vi "6.0.0_Pump Motor Test.vi"(6 ".batCMD":T1={"Brush_ADC.bat"="Brush_ADC.bat", "Get Release Version.bat"="Get Release Version.bat", "Getting Software  Version.bat"="Getting Software  Version.bat", "Pump_ADC.bat"="Pump_ADC.bat", "Starting  Pump Motor.bat"="Starting  Pump Motor.bat", "Starting  Test Mode.bat"="Starting  Test Mode.bat", "Starting Brush Motor 1.bat"="Starting Brush Motor 1.bat", "Starting Brush Motor 2.bat"="Starting Brush Motor 2.bat", "Starting Brush Motor 3.bat"="Starting Brush Motor 3.bat", "Starting LED Test.bat"="Starting LED Test.bat", "Stopping  Brush Motor.bat"="Stopping  Brush Motor.bat", "Stopping  Pump Motor.bat"="Stopping  Pump Motor.bat", "Stopping  Test Mode.bat"="Stopping  Test Mode.bat", "Starting Self Test.bat"="Starting Self Test.bat", "Software Reset.bat"="Software Reset.bat", "Get HW version.bat"="Get HW version.bat", "Read PMIC status.bat"="Read PMIC status.bat", "SC IMU Data Streaming.bat"="SC IMU Data Streaming.bat"}, 7 "Data in":T2, 8 "error in (no error)":errorcluster, 9 "AllControls In":T3, 10 "?":T4, 11 "Message Queue out":T5) -> (0 "error out":errorcluster, 1 "Flow":string, 2 "Data":T4, 3 "Message Queue Out":T5, 5 "Data out":T2)   [LabVIEW 2017]
uses:
  Depends/AMC/subVIs/TypeDefs/amc_Message Queue.ctl
  Depends/AMC/subVIs/TypeDefs/amc_Message.ctl
  Depends/Tools/Keyed Array/Tools_KeyedArray KeyedArray.ctl
  Ctrls/Data.ctl
  Ctrls/AllControls.ctl
  Ctrls/CSV_Data.ctl
  0516/X682 Chassis Connectivity Tester Program/Ctrls/682_cmd.ctl
  <instrlib>/GPP/GPP.lvlib
types:
  T1 = typedef "682_cmd.ctl" = cluster{"Brush_ADC.bat":string, "Get Release Version.bat":string, "Getting Software  Version.bat":string, "Pump_ADC.bat":string, "Starting  Pump Motor.bat":string, "Starting  Test Mode.bat":string, "Starting Brush Motor 1.bat":string, "Starting Brush Motor 2.bat":string, "Starting Brush Motor 3.bat":string, "Starting LED Test.bat":string, "Stopping  Brush Motor.bat":string, "Stopping  Pump Motor.bat":string, "Stopping  Test Mode.bat":string, "Starting Self Test.bat":string, "Software Reset.bat":string, "Get HW version.bat":string, "Read PMIC status.bat":string, "SC IMU Data Streaming.bat":string}
  T2 = typedef "CSV_Data.ctl" = cluster{"Initialisation":cluster{"LMT - Connect UUT (con COM)":string, "LMT - Software Version (rrel)":string, "LMT - Write SKU file (wskuc)":string, "LMT - SKU file name":string, "Connect UUT DDM":string, "Read DDM EOL Timestamp - Mode":string, "Read DDM EOL Timestamp - Timestamp":string, "Read DDM EOL Timestamp - Rig ID":string, "Read DDM EOL Timestamp - Passmark ID":string, "Read DDM EOL Timestamp - Passmark Rev":string, "Software Version before flashing":string, "Read Hardware Serial":string, "UUT DDM SN":string, "Compare DDM SN with MES SN":string, "Backup PCBA Calibration EEPROM Response - CAL":string, "Flash Firmware Version":string, "Check SW Version":string, "Read DDM SW Version after flashing":string, "Set SKU Config":string, "Ready Status":string, "Set Device Mode to EOL":string, "DDM Parameter - Voltage":string, "DDM Parameter - Current":string, "DDM Parameter - Power":string, "DDM Parameter - Speed":string, "DDM Parameter - Pressure":string, "Tester Parameter - Voltage":string, "Tester Parameter - Current":string, "Tester Parameter - Power":string, "Tester Parameter - Ambient Pressure":string, "Tester Parameter - Ambient Temperature":string, "Calculated Parameter - DDM Pressure Corrected":string, "Calculated Parameter - DDM Real Power":string, "Calculated Parameter - Delta V":string}, "BEMF_Calibration":cluster{"Calibration Result - eol_cold_bemf_temp":string, "DDM Ambient Temp":string, "Restriction Plate Diameter":string, "Calibration Result - eol_bemf_mp_cold_coef_a":string, "Calibration Result - eol_bemf_mp_cold_coef_b":string, "Calibration Result - eol_bemf_mp_cold_coef_c":string, "Calibration Result - eol_bemf_lsi_cold_ref_coeffs":string, "Get - Calibration Result - eol_bemf_lsi_speed":string, "Get - Calibration Result - eol_bemf_lsi_integral_0":string, "Calibration Result - eol_bemf_lsi_integral_1":string, "Get - Calibration Result - eol_bemf_lsi_integral_2":string, "Get - Calibration Result - eol_cold_bemf":string, "Get - Calibration Result - eol_cold_bemf_fisf":string, "Finalise Calibration":string, "Compare -Calibration Result - eol_cold_bemf":string, "Compare -Calibration Result - eol_cold_bemf_fisf":string}, "ECO":cluster{"Reset Power Tune":string, "Reset BEMF FISF Calibration":string, "Restriction Plate Diameter":string, "ECO - Stabilisation Time":string, "ECO - DDM Parameter - Voltage":string, "ECO - DDM Parameter - Current":string, "ECO - DDM Parameter - Power":string, "ECO - DDM Parameter - Measured Power":string, "ECO - DDM Parameter - Speed":string, "ECO - DDM Parameter - Pressure":string, "ECO - Tester Parameter - Voltage":string, "ECO - Tester Parameter - Current":string, "ECO - Tester Parameter - Power":string, "ECO - Tester Parameter - Ambient Pressure":string, "ECO - Tester Parameter - Ambient Temperature":string, "ECO - Tester Parameter - Ambient Humidity":string, "ECO - Calculated Parameter - DDM Pressure Corrected":string, "ECO - Calculated Parameter - DDM Real Power":string, "ECO - Calculated Parameter - Delta V":string, "ECO - Calculated Parameter - Flowrate":string, "ECO - Calculated Parameter - Airwatt":string, "ECO - Formula":string, "PT ECO - Power Tune Mode Status":string}, "BOOST":cluster{"Restriction Plate Diameter":string, "BOOST - Stabilisation Time":string, "BOOST - DDM Parameter - Voltage":string, "BOOST - DDM Parameter - Current":string, "BOOST - DDM Parameter - Power":string, "BOOST - DDM Parameter - Measured Power":string, "BOOST - DDM Parameter - Speed":string, "BOOST - DDM Parameter - Pressure":string, "BOOST - Tester Parameter - Voltage":string, "BOOST - Tester Parameter - Current":string, "BOOST - Tester Parameter - Power":string, "BOOST - Tester Parameter - Ambient Pressure":string, "BOOST - Tester Parameter - Ambient Temperature":string, "BOOST - Tester Parameter - Ambient Humidity":string, "BOOST - Calculated Parameter - DDM Pressure Corrected":string, "BOOST - Calculated Parameter - DDM Real Power":string, "BOOST - Calculated Parameter - Delta V":string, "BOOST - Calculated Parameter - Flowrate":string, "BOOST - Calculated Parameter - Airwatt":string, "BOOST - Get AM Presence":string, "Air Muscle Turn Off Status":string, "BOOST - Air Muscle Calculated Parameter - Airwatt B":string, "BOOST - Air Muscle Calculate Airwatt Delta":string, "PT BOOST - Power Tune Mode Status":string, "Finalise Calibration":string, "ECO - Get AW Calibration value":string, "BOOST - Get AW Calibration value":string}, "MAX":cluster{"Restriction Plate Diameter":string, "MAX - Stabilisation Time":string, "Get Average Delta Tmag (LSIdelta_FISFdelta_LSItmag_FISFtmag_IIRtmag)":string, "Get Average Delta Tmag FISF":string, "MAX - DDM Parameter - Voltage":string, "MAX - DDM Parameter - Current":string, "MAX - DDM Parameter - Power":string, "MAX - DDM Parameter - Measured Power":string, "MAX - DDM Parameter - Speed":string, "MAX - DDM Parameter - Pressure":string, "MAX - Tester Parameter - Voltage":string, "MAX - Tester Parameter - Current":string, "MAX - Tester Parameter - Power":string, "MAX - Tester Parameter - Ambient Pressure":string, "MAX - Tester Parameter - Ambient Temperature":string, "MAX - Tester Parameter - Ambient Humidity":string, "MAX - Calculated Parameter - DDM Pressure Corrected":string, "MAX - Calculated Parameter - DDM Real Power":string, "MAX - Calculated Parameter - Delta V":string, "MAX - Calculated Parameter - Flowrate":string, "MAX - Calculated Parameter - Airwatt":string, "MAX_FISF_Check_Average_Delta_Tmag":string, "MAX - FISF - BEMF Finetune Result":string, "MAX tune - Delta P1":string, "MAX tune - Calculated Parameter - Airwatt":string, "Calculate Delta Airwatts - MAX finetune - Delta P2":string, "MAX finetune - DDM Parameter - Voltage":string, "MAX finetune - DDM Parameter - Current":string, "MAX finetune - DDM Parameter - Power":string, "MAX finetune - DDM Parameter - Measured Power":string, "MAX finetune - DDM Parameter - Speed":string, "MAX finetune - DDM Parameter - Pressure":string, "MAX finetune - Tester Parameter - Voltage":string, "MAX finetune - Tester Parameter - Current":string, "MAX finetune - Tester Parameter - Power":string, "MAX finetune - Tester Parameter - Ambient Pressure":string, "MAX finetune - Tester Parameter - Ambient Temperature":string, "MAX finetune - Tester Parameter - Ambient Humidity":string, "MAX finetune - Calculated Parameter - DDM Pressure Corrected":string, "MAX finetune - Calculated Parameter - DDM Real Power":string, "MAX finetune - Calculated Parameter - Delta V":string, "MAX finetune - Calculated Parameter - Flowrate":string, "MAX finetune - Calculated Parameter - Airwatt":string, "Check Derate Result":string, "Delta Tmag FISF":string, "Get Hot BEMF Result":string, "Calculate delta Pressure":string, "Finalise Calibration":string, "Calculate & Check Delta BEMF":string, "Delta P Airwatts Value":string}, "LL":cluster{"DDM Ambient Temp":string, "Restriction Plate Diameter":string, "LL - DDM Parameter - Voltage":string, "LL - DDM Parameter - Current":string, "LL - DDM Parameter - Power":string, "LL - DDM Parameter - Measured Power":string, "LL - DDM Parameter - Speed":string, "LL - DDM Parameter - Pressure":string, "LL - Tester Parameter - Voltage":string, "LL - Tester Parameter - Current":string, "LL - Tester Parameter - Power":string, "LL - DDM Real Power":string, "LL - Calibrate Task Detect LL":string}, "HL":cluster{"HL - DDM Parameter - Voltage":string, "HL - DDM Parameter - Current":string, "HL - DDM Parameter - Power":string, "HL - DDM Parameter - Measured Power":string, "HL - DDM Parameter - Speed":string, "HL - DDM Parameter - Pressure":string, "HL - Tester Parameter - Voltage":string, "HL - Tester Parameter - Current":string, "HL - Tester Parameter - Power":string, "HL - DDM Real Power":string, "HL - Calibrate Task Detect HL":string}, "LH":cluster{"Restriction Plate Diameter":string, "LH - DDM Parameter - Voltage":string, "LH - DDM Parameter - Current":string, "LH - DDM Parameter - Power":string, "LH - DDM Parameter - Measured Power":string, "LH - DDM Parameter - Speed":string, "LH - DDM Parameter - Pressure":string, "LH - Tester Parameter - Voltage":string, "LH - Tester Parameter - Current":string, "LH - Tester Parameter - Power":string, "LH - DDM Real Power":string, "LH - Calibrate Task Detect LH":string}, "HH":cluster{"HH - DDM Parameter - Voltage":string, "HH - DDM Parameter - Current":string, "HH - DDM Parameter - Power":string, "HH - DDM Parameter - Measured Power":string, "HH - DDM Parameter - Speed":string, "HH - DDM Parameter - Pressure":string, "HH - Tester Parameter - Voltage":string, "HH - Tester Parameter - Current":string, "HH - Tester Parameter - Power":string, "HH - DDM Real Power":string, "HH - Calibrate Task Detect HH":string}, "Inlet Blockage Calibration":cluster{"Inlet Blockage Calibration - DDM Parameter - Voltage":string, "Inlet Blockage Calibration - DDM Parameter - Current":string, "Inlet Blockage Calibration - DDM Parameter - Power":string, "Inlet Blockage Calibration - DDM Parameter - Measured Power":string, "Inlet Blockage Calibration - DDM Parameter - Speed":string, "Inlet Blockage Calibration - DDM Parameter - Pressure":string, "Inlet Blockage Calibration - Tester Parameter - Voltage":string, "Inlet Blockage Calibration - Tester Parameter - Current":string, "Inlet Blockage Calibration - Tester Parameter - Power":string, "Inlet Blockage Calibration - DDM Real Power":string, "Calibration Inlet Blockage_E":string, "Finalise Calibration":string, "Get Task Detect LL":string, "Get Task Detect HL":string, "Get Task Detect LH":string, "Get Task Detect HH":string, "Calibration Inlet Blockage":string, "Calibration eol cold bemf temp":string}, "GOOD":cluster{"GOOD UNIT - Clear EEPROM Error Log":string, "GOOD UNIT - Write Product Timestamp - Mode":string, "GOOD UNIT - Write Product Timestamp - Timestamp":string, "GOOD UNIT - Write Product Timestamp - Rig ID":string, "GOOD UNIT - Write Product Timestamp - Passmark ID":string, "GOOD UNIT - Write Product Timestamp - Passmark Rev":string, "GOOD UNIT - Set Device Mode to PROD":string, "GOOD UNIT - Backup PCBA Calibration EEPROM Response":string, "GOOD UNIT - Check Security Bit":string, "GOOD UNIT - Set Calibration Lock":string, "GOOD UNIT - Get_Calibration_Lock":string, "GOOD UNIT - Disconnect UUT":string}, "NG":cluster{"NG UNIT - Read NVM Error":string, "NG UNIT - Set Device Mode to FCT":string, "NG UNIT - Backup PCBA Calibration EEPROM Response - CAL":string, "NG UNIT - Backup PCBA Calibration EEPROM Response - ERROR":string, "NG UNIT - Backup PCBA Calibration EEPROM Response - USAGE":string, "NG UNIT - Disconnect UUT":string}, "SN":string, "Table":string[][], "Count":cluster{"Total":i32, "OK":i32, "NG":i32, "Yield":dbl}, "Start Time":timestamp, "daemon reference":refnum<k5>, "CT":dbl, "Config":string[][], "OK/NG":bool, "Station ID":string, "MES DDM SN":string, "MES PCBA SN":string, "Retest":string, "Lux":string, "Initialisation_Status":cluster{"LMT - Connect UUT (con COM)":string, "LMT - Software Version (rrel)":string, "LMT - Write SKU file (wskuc)":string, "LMT - SKU file name":string, "Connect UUT DDM":string, "Read DDM EOL Timestamp - Mode":string, "Read DDM EOL Timestamp - Timestamp":string, "Read DDM EOL Timestamp - Rig ID":string, "Read DDM EOL Timestamp - Passmark ID":string, "Read DDM EOL Timestamp - Passmark Rev":string, "Software Version before flashing":string, "Read Hardware Serial":string, "UUT DDM SN":string, "Compare DDM SN with MES SN":string, "Backup PCBA Calibration EEPROM Response - CAL":string, "Flash Firmware Version":string, "Check SW Version":string, "Read DDM SW Version after flashing":string, "Set SKU Config":string, "Ready Status":string, "Set Device Mode to EOL":string, "DDM Parameter - Voltage":string, "DDM Parameter - Current":string, "DDM Parameter - Power":string, "DDM Parameter - Speed":string, "DDM Parameter - Pressure":string, "Tester Parameter - Voltage":string, "Tester Parameter - Current":string, "Tester Parameter - Power":string, "Tester Parameter - Ambient Pressure":string, "Tester Parameter - Ambient Temperature":string, "Calculated Parameter - DDM Pressure Corrected":string, "Calculated Parameter - DDM Real Power":string, "Calculated Parameter - Delta V":string}, "BEMF_Calibration_Status":cluster{"Calibration Result - eol_cold_bemf_temp":string, "DDM Ambient Temp":string, "Restriction Plate Diameter":string, "Calibration Result - eol_bemf_mp_cold_coef_a":string, "Calibration Result - eol_bemf_mp_cold_coef_b":string, "Calibration Result - eol_bemf_mp_cold_coef_c":string, "Calibration Result - eol_bemf_lsi_cold_ref_coeffs":string, "Get - Calibration Result - eol_bemf_lsi_speed":string, "Get - Calibration Result - eol_bemf_lsi_integral_0":string, "Calibration Result - eol_bemf_lsi_integral_1":string, "Get - Calibration Result - eol_bemf_lsi_integral_2":string, "Get - Calibration Result - eol_cold_bemf":string, "Get - Calibration Result - eol_cold_bemf_fisf":string, "Finalise Calibration":string, "Compare -Calibration Result - eol_cold_bemf":string, "Compare -Calibration Result - eol_cold_bemf_fisf":string}, "ECO_Status":cluster{"Reset Power Tune":string, "Reset BEMF FISF Calibration":string, "Restriction Plate Diameter":string, "ECO - Stabilisation Time":string, "ECO - DDM Parameter - Voltage":string, "ECO - DDM Parameter - Current":string, "ECO - DDM Parameter - Power":string, "ECO - DDM Parameter - Measured Power":string, "ECO - DDM Parameter - Speed":string, "ECO - DDM Parameter - Pressure":string, "ECO - Tester Parameter - Voltage":string, "ECO - Tester Parameter - Current":string, "ECO - Tester Parameter - Power":string, "ECO - Tester Parameter - Ambient Pressure":string, "ECO - Tester Parameter - Ambient Temperature":string, "ECO - Tester Parameter - Ambient Humidity":string, "ECO - Calculated Parameter - DDM Pressure Corrected":string, "ECO - Calculated Parameter - DDM Real Power":string, "ECO - Calculated Parameter - Delta V":string, "ECO - Calculated Parameter - Flowrate":string, "ECO - Calculated Parameter - Airwatt":string, "ECO - Formula":string, "PT ECO - Power Tune Mode Status":string}, "BOOST_Status":cluster{"Restriction Plate Diameter":string, "BOOST - Stabilisation Time":string, "BOOST - DDM Parameter - Voltage":string, "BOOST - DDM Parameter - Current":string, "BOOST - DDM Parameter - Power":string, "BOOST - DDM Parameter - Measured Power":string, "BOOST - DDM Parameter - Speed":string, "BOOST - DDM Parameter - Pressure":string, "BOOST - Tester Parameter - Voltage":string, "BOOST - Tester Parameter - Current":string, "BOOST - Tester Parameter - Power":string, "BOOST - Tester Parameter - Ambient Pressure":string, "BOOST - Tester Parameter - Ambient Temperature":string, "BOOST - Tester Parameter - Ambient Humidity":string, "BOOST - Calculated Parameter - DDM Pressure Corrected":string, "BOOST - Calculated Parameter - DDM Real Power":string, "BOOST - Calculated Parameter - Delta V":string, "BOOST - Calculated Parameter - Flowrate":string, "BOOST - Calculated Parameter - Airwatt":string, "BOOST - Get AM Presence":string, "Air Muscle Turn Off Status":string, "BOOST - Air Muscle Calculated Parameter - Airwatt B":string, "BOOST - Air Muscle Calculate Airwatt Delta":string, "PT BOOST - Power Tune Mode Status":string, "Finalise Calibration":string, "ECO - Get AW Calibration value":string, "BOOST - Get AW Calibration value":string}, "MAX_Status":cluster{"Restriction Plate Diameter":string, "MAX - Stabilisation Time":string, "Get Average Delta Tmag (LSIdelta_FISFdelta_LSItmag_FISFtmag_IIRtmag)":string, "Get Average Delta Tmag FISF":string, "MAX - DDM Parameter - Voltage":string, "MAX - DDM Parameter - Current":string, "MAX - DDM Parameter - Power":string, "MAX - DDM Parameter - Measured Power":string, "MAX - DDM Parameter - Speed":string, "MAX - DDM Parameter - Pressure":string, "MAX - Tester Parameter - Voltage":string, "MAX - Tester Parameter - Current":string, "MAX - Tester Parameter - Power":string, "MAX - Tester Parameter - Ambient Pressure":string, "MAX - Tester Parameter - Ambient Temperature":string, "MAX - Tester Parameter - Ambient Humidity":string, "MAX - Calculated Parameter - DDM Pressure Corrected":string, "MAX - Calculated Parameter - DDM Real Power":string, "MAX - Calculated Parameter - Delta V":string, "MAX - Calculated Parameter - Flowrate":string, "MAX - Calculated Parameter - Airwatt":string, "MAX_FISF_Check_Average_Delta_Tmag":string, "MAX - FISF - BEMF Finetune Result":string, "MAX tune - Delta P1":string, "MAX tune - Calculated Parameter - Airwatt":string, "Calculate Delta Airwatts - MAX finetune - Delta P2":string, "MAX finetune - DDM Parameter - Voltage":string, "MAX finetune - DDM Parameter - Current":string, "MAX finetune - DDM Parameter - Power":string, "MAX finetune - DDM Parameter - Measured Power":string, "MAX finetune - DDM Parameter - Speed":string, "MAX finetune - DDM Parameter - Pressure":string, "MAX finetune - Tester Parameter - Voltage":string, "MAX finetune - Tester Parameter - Current":string, "MAX finetune - Tester Parameter - Power":string, "MAX finetune - Tester Parameter - Ambient Pressure":string, "MAX finetune - Tester Parameter - Ambient Temperature":string, "MAX finetune - Tester Parameter - Ambient Humidity":string, "MAX finetune - Calculated Parameter - DDM Pressure Corrected":string, "MAX finetune - Calculated Parameter - DDM Real Power":string, "MAX finetune - Calculated Parameter - Delta V":string, "MAX finetune - Calculated Parameter - Flowrate":string, "MAX finetune - Calculated Parameter - Airwatt":string, "Check Derate Result":string, "Delta Tmag FISF":string, "Get Hot BEMF Result":string, "Calculate delta Pressure":string, "Finalise Calibration":string, "Calculate & Check Delta BEMF":string, "Delta P Airwatts Value":string}, "LL_Status":cluster{"DDM Ambient Temp":string, "Restriction Plate Diameter":string, "LL - DDM Parameter - Voltage":string, "LL - DDM Parameter - Current":string, "LL - DDM Parameter - Power":string, "LL - DDM Parameter - Measured Power":string, "LL - DDM Parameter - Speed":string, "LL - DDM Parameter - Pressure":string, "LL - Tester Parameter - Voltage":string, "LL - Tester Parameter - Current":string, "LL - Tester Parameter - Power":string, "LL - DDM Real Power":string, "LL - Calibrate Task Detect LL":string}, "HL_Status":cluster{"HL - DDM Parameter - Voltage":string, "HL - DDM Parameter - Current":string, "HL - DDM Parameter - Power":string, "HL - DDM Parameter - Measured Power":string, "HL - DDM Parameter - Speed":string, "HL - DDM Parameter - Pressure":string, "HL - Tester Parameter - Voltage":string, "HL - Tester Parameter - Current":string, "HL - Tester Parameter - Power":string, "HL - DDM Real Power":string, "HL - Calibrate Task Detect HL":string}, "LH_Status":cluster{"Restriction Plate Diameter":string, "LH - DDM Parameter - Voltage":string, "LH - DDM Parameter - Current":string, "LH - DDM Parameter - Power":string, "LH - DDM Parameter - Measured Power":string, "LH - DDM Parameter - Speed":string, "LH - DDM Parameter - Pressure":string, "LH - Tester Parameter - Voltage":string, "LH - Tester Parameter - Current":string, "LH - Tester Parameter - Power":string, "LH - DDM Real Power":string, "LH - Calibrate Task Detect LH":string}, "HH_Status":cluster{"HH - DDM Parameter - Voltage":string, "HH - DDM Parameter - Current":string, "HH - DDM Parameter - Power":string, "HH - DDM Parameter - Measured Power":string, "HH - DDM Parameter - Speed":string, "HH - DDM Parameter - Pressure":string, "HH - Tester Parameter - Voltage":string, "HH - Tester Parameter - Current":string, "HH - Tester Parameter - Power":string, "HH - DDM Real Power":string, "HH - Calibrate Task Detect HH":string}, "Inlet Blockage Calibration_Status":cluster{"Inlet Blockage Calibration - DDM Parameter - Voltage":string, "Inlet Blockage Calibration - DDM Parameter - Current":string, "Inlet Blockage Calibration - DDM Parameter - Power":string, "Inlet Blockage Calibration - DDM Parameter - Measured Power":string, "Inlet Blockage Calibration - DDM Parameter - Speed":string, "Inlet Blockage Calibration - DDM Parameter - Pressure":string, "Inlet Blockage Calibration - Tester Parameter - Voltage":string, "Inlet Blockage Calibration - Tester Parameter - Current":string, "Inlet Blockage Calibration - Tester Parameter - Power":string, "Inlet Blockage Calibration - DDM Real Power":string, "Calibration Inlet Blockage_E":string, "Finalise Calibration":string, "Get Task Detect LL":string, "Get Task Detect HL":string, "Get Task Detect LH":string, "Get Task Detect HH":string, "Calibration Inlet Blockage":string, "Calibration eol cold bemf temp":string}, "GOOD_Status":cluster{"GOOD UNIT - Clear EEPROM Error Log":string, "GOOD UNIT - Write Product Timestamp - Mode":string, "GOOD UNIT - Write Product Timestamp - Timestamp":string, "GOOD UNIT - Write Product Timestamp - Rig ID":string, "GOOD UNIT - Write Product Timestamp - Passmark ID":string, "GOOD UNIT - Write Product Timestamp - Passmark Rev":string, "GOOD UNIT - Set Device Mode to PROD":string, "GOOD UNIT - Backup PCBA Calibration EEPROM Response":string, "GOOD UNIT - Check Security Bit":string, "GOOD UNIT - Set Calibration Lock":string, "GOOD UNIT - Get_Calibration_Lock":string, "GOOD UNIT - Disconnect UUT":string}, "NG_Status":cluster{"NG UNIT - Read NVM Error":string, "NG UNIT - Set Device Mode to FCT":string, "NG UNIT - Backup PCBA Calibration EEPROM Response - CAL":string, "NG UNIT - Backup PCBA Calibration EEPROM Response - ERROR":string, "NG UNIT - Backup PCBA Calibration EEPROM Response - USAGE":string, "NG UNIT - Disconnect UUT":string}, "SKU":string, "Plate_Diameter":string, "Alarm":string}
  T3 = typedef "AllControls.ctl" = cluster{"MainVI":refnum<vi>, "AlarmInfo":refnum<vi>, "Log":refnum<vi>, "Current CT":refnum<vi>, "ProductID":refnum<vi>, "Device state":refnum<vi>, "MES":refnum<vi>, "mode":refnum<vi>, "TestInfo":refnum<vi>, "SubPnl":refnum<vi>, "Table":refnum<vi>, "MES bool":refnum<vi>, "TestMode":refnum<vi>, "Recipe":refnum<vi>, "Fail resume":refnum<vi>, "LogIn":refnum<vi>, "Start":refnum<vi>, "Maintenance":refnum<vi>, "Stop":refnum<vi>, "Exit":refnum<vi>}
  T4 = typedef "Data.ctl" = cluster{"Initialisation":cluster{"DDM_Parameter":dbl[], "DDM_Parameter_status":bool[], "Get_Tester_Parameter":dbl[], "Get_Tester_Parameter_status":bool[], "Cal_Tester_Parameter":dbl[], "Cal_Tester_Parameter_status":bool[], "sw_version_before_status":bool, "sw_version_after_status":bool, "Set_SKU_Config_With_LMT_status":bool, "FCT_timestamp_status":bool, "LMT_Connect_to_UUT_status":bool}, "BEMF_Calibration":cluster{"Read_ambient_temperature":dbl, "Calibration_Vaule":dbl[], "Calibration_Vaule _B":dbl[], "Calibration_Vaule_status":bool[], "Calibration_Vaule_B_status":bool[]}, "ECO":cluster{"DDM_Parameter":dbl[], "DDM_Parameter_status":bool[], "Get_Tester_Parameter":dbl[], "Get_Tester_Parameter_status":bool[], "Cal_Tester_Parameter":dbl[], "Cal_Tester_Parameter_status":bool[], "DDM_Parameter_after_power_tune":dbl[], "Get_Tester_Parameter_after_power_tune":dbl[], "Cal_Tester_Parameter_after_power_tune":dbl[], "Cal_Tester_Parameter_after_power_tune_status":bool[], "Delta_P":dbl}, "BOOST":cluster{"DDM_Parameter":dbl[], "DDM_Parameter_status":bool[], "Get_Tester_Parameter":dbl[], "Get_Tester_Parameter_status":bool[], "Cal_Tester_Parameter":dbl[], "Cal_Tester_Parameter_status":bool[], "DDM_Parameter_after_power_tune":dbl[], "Get_Tester_Parameter_after_power_tune":dbl[], "Cal_Tester_Parameter_after_power_tune":dbl[], "Cal_Tester_Parameter_after_power_tune_status":bool[], "airwatts_am_off":dbl, "AW_Delta_(AM_on_and_off)":dbl, "AW_Delta_(AM_on_and_off)_Status":bool, "Delta_P":dbl}, "MAX":cluster{"Average_Tmag_Data":cluster{"LSI Delta in degC":dbl, "FISF Delta in degc":dbl, "LSI Tmag in degC":dbl, "Fisf Tmag in degC":dbl, "IIR Tmag in degC":dbl}, "DDM_Parameter":dbl[], "DDM_Parameter_status":bool[], "Get_Tester_Parameter":dbl[], "Get_Tester_Parameter_status":bool[], "Cal_Tester_Parameter":dbl[], "BEMF_Finetune":cluster{"eol_bemf_mp_cold_coef_c":dbl, "eol_cold_bemf_fisf_offset":dbl}, "AW_Tune":cluster{"delta_P1":dbl, "delta_P_Setting":dbl}, "DDM_Parameter_after_Airwatts_Tune":dbl[], "Get_Tester_Parameter_after_Airwatts_Tune":dbl[], "Cal_Tester_Parameter_after_Airwatts_Tune":dbl[], "DDM_Parameter_after_Airwatts_Finetune":dbl[], "Get_Tester_Parameter_after_Airwatts_Finetune":dbl[], "Cal_Tester_Parameter_after_Airwatts_Finetune":dbl[], "AW_Finetune":cluster{"delta_P2":dbl, "delta_P_Setting":dbl}, "Delta_Tmag_after_tune":cluster{"LSI Delta in degC":dbl, "FISF Delta in degc":dbl, "LSI Tmag in degC":dbl, "Fisf Tmag in degC":dbl, "IIR Tmag in degC":dbl}, "Hot Bemf in mV":dbl, "DDM_Pressure":dbl, "Delta_Pressure":dbl, " Cold Bemf in mV":dbl, " delta Bemf":dbl, " delta p":dbl, "Delta_Pressure_status":bool, " delta Bemf_status":bool, "LSI Delta in degC_status":bool, "FISF Delta in degc_status":bool, "Max_check_derate_status_status":bool, "Average_All_data":dbl[][], "Average_Tmag_Data_status":bool[], "Average_Tmag_Data_after_tune_status":bool[], "Cal_Tester_Parameter_status":bool[], "Cal_Tester_Parameter_status_after_Airwatts_Tune":bool[], "Cal_Tester_Parameter_status_after_Airwatts_FineTune":bool[]}, "Task_Detect_Calib":cluster{"LL":cluster{"DDM_Parameter":dbl[], "DDM_Parameter_status":bool[], "Get_Tester_Parameter":dbl[], "Get_Tester_Parameter_status":bool[], "Set_task_detect_A":dbl, "Set_task_detect_A_Status":bool}, "HL":cluster{"DDM_Parameter":dbl[], "DDM_Parameter_status":bool[], "Get_Tester_Parameter":dbl[], "Get_Tester_Parameter_status":bool[], "Set_task_detect_B":dbl, "Set_task_detect_B_Status":bool}, "LH":cluster{"DDM_Parameter":dbl[], "DDM_Parameter_status":bool[], "Get_Tester_Parameter":dbl[], "Get_Tester_Parameter_status":bool[], "Set_task_detect_C":dbl, "Set_task_detect_C_Status":bool}, "HH":cluster{"DDM_Parameter":dbl[], "DDM_Parameter_status":bool[], "Get_Tester_Parameter":dbl[], "Get_Tester_Parameter_status":bool[], "Set_task_detect_D":dbl, "Read_and_check_calibration_Status":bool[], "Set_task_detect_D_Status":bool}, "Get_eol_inlet_blockage_E":dbl, "Calib_vaule":cluster{"Get_task_detect_LL":dbl, "Get_task_detect_HL":dbl, "Get_task_detect_LH":dbl, "Get_task_detect_HH":dbl, "eol_inlet_blockage":dbl, "eol_code_bemf_temp":dbl}, "calibrated temp":dbl, "Inlet_Blockage_Calibration":cluster{"DDM_Parameter":dbl[], "DDM_Parameter_status":bool[], "Get_Tester_Parameter":dbl[], "Get_Tester_Parameter_status":bool[]}, "Get_eol_inlet_blockage_E_Status":bool}, "good":cluster{"Write_Product_TS":cluster{"TIMESTAMP":i64, "RIG_ID":i64, "PASSMARK_ID":i64, "PASSMARK_REV":i64}, "Read_Product_TS":cluster{"TIMESTAMP":i64, "RIG_ID":i64, "PASSMARK_ID":i64, "PASSMARK_REV":i64}, "Good_Check_Secuity_Bit_Stauts":bool}}
  T5 = typedef "amc_Message Queue.ctl" = refnum<queue>
  T6 = typedef "HD Config.ctl" = cluster{" PC":cluster{"PC Address":u8[], "PC Port":i32}, "FCO":cluster{"COM":refnum<visa-resource-name>, "Baudrate":u32}, "DC Power ":cluster{"COM":refnum<visa-resource-name>, "Baudrate":u32}, "PW3336":cluster{"COM":refnum<visa-resource-name>, "Baudrate":u32}, "Lefoo":cluster{"COM":refnum<visa-resource-name>, "Baudrate":u32}, "Tempt&Hum":cluster{"COM":refnum<visa-resource-name>, "Baudrate":u32}, "DIPC":cluster{"COM":refnum<visa-resource-name>}, "Daemon":cluster{"IP Address":string, "Port":u16, "Retry":u16}, "URAT":cluster{"COM":refnum<visa-resource-name>, "Baudrate":u32}, "Fail_resume_mode":bool, "GRR":bool}
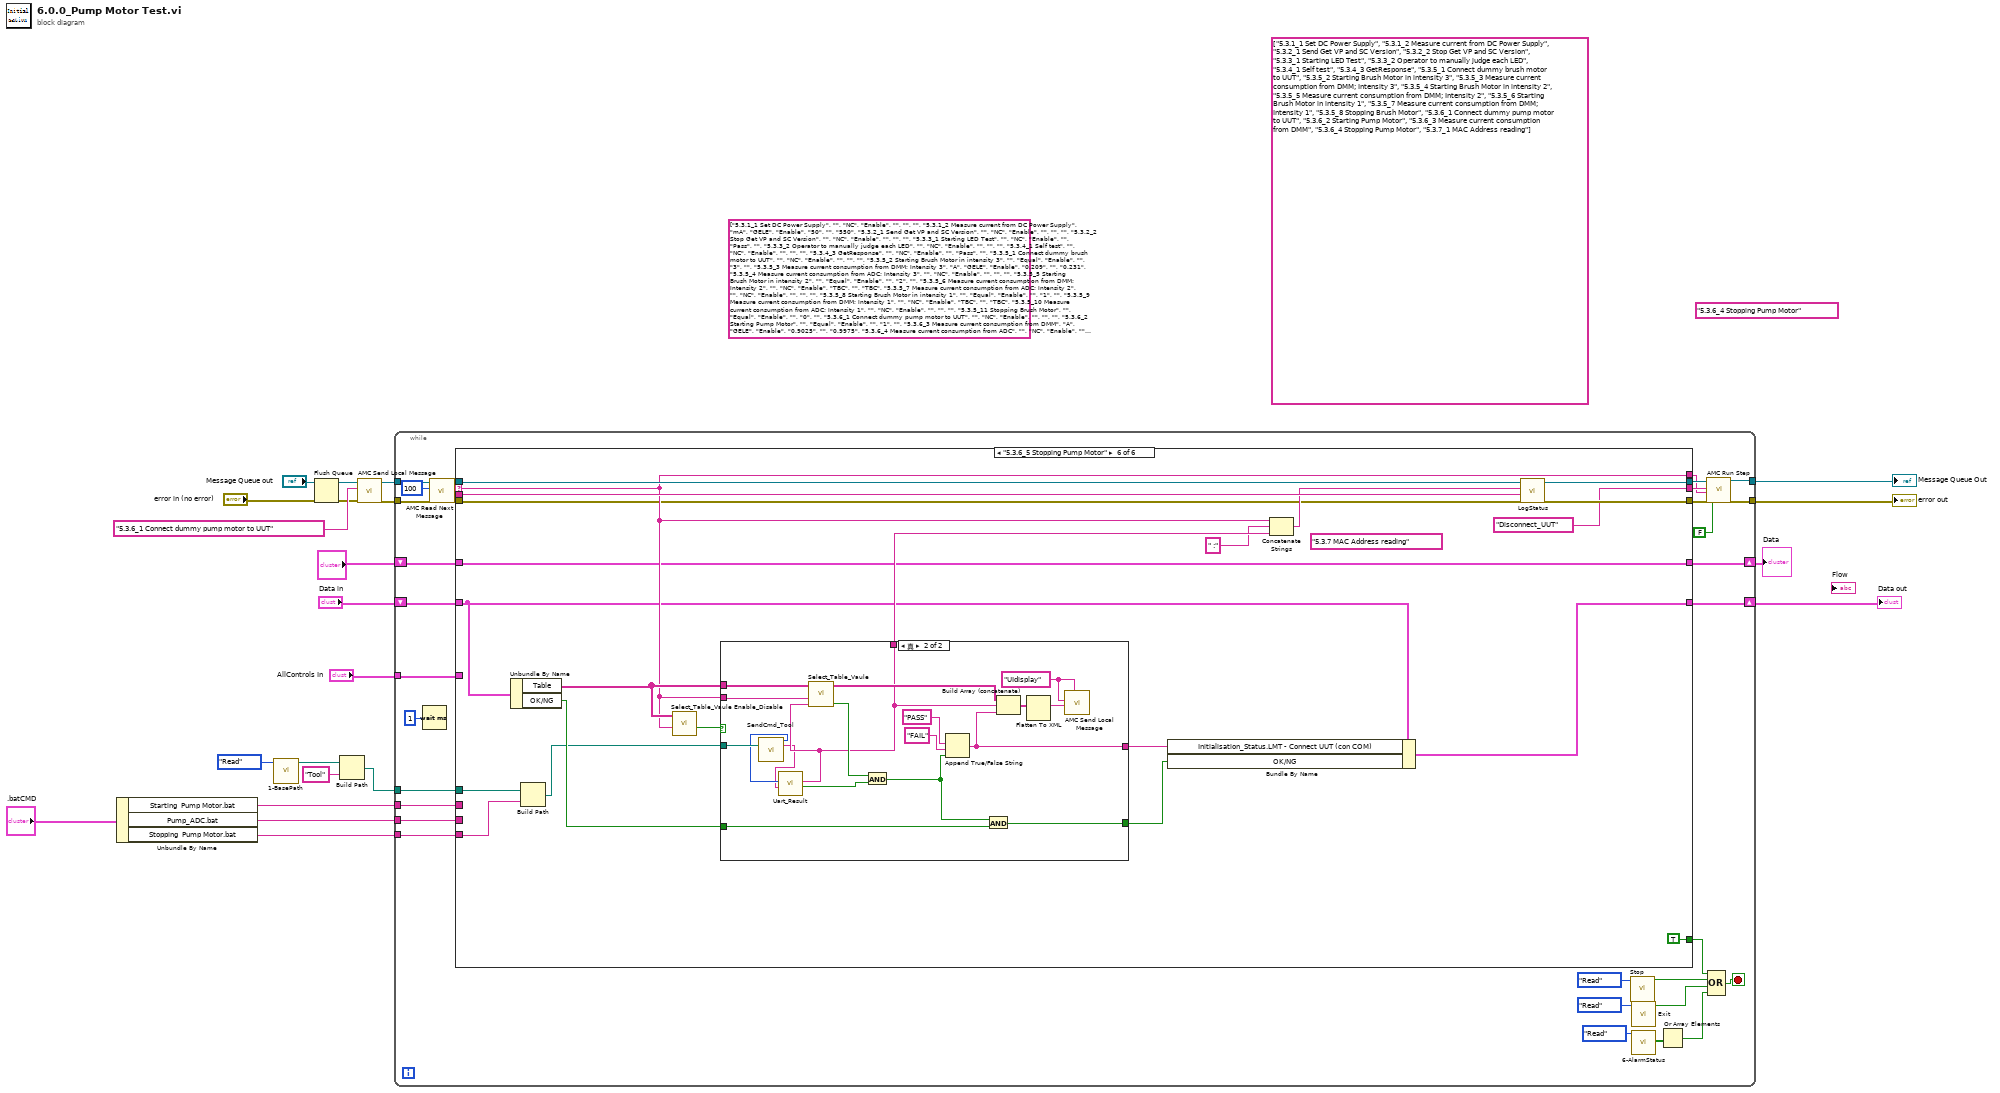
[diagram p0: block diagram]
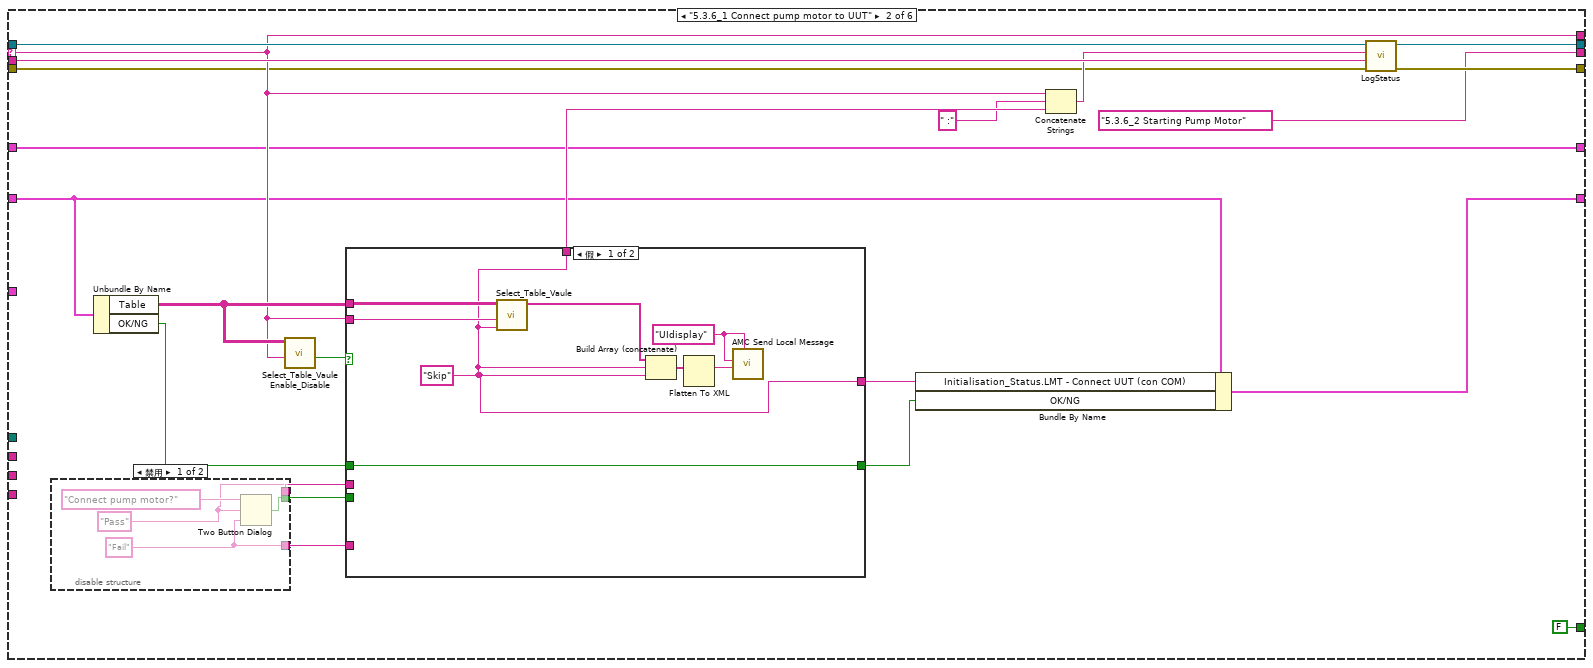
[diagram p3: hidden frame]
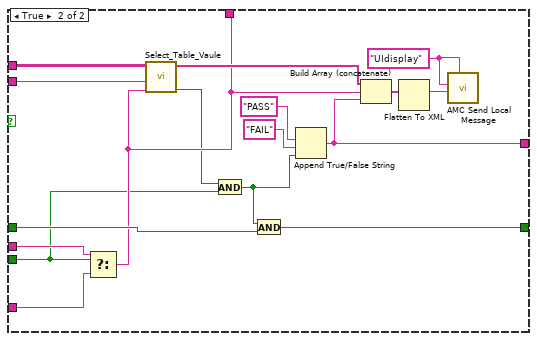
[diagram p5: hidden frame]
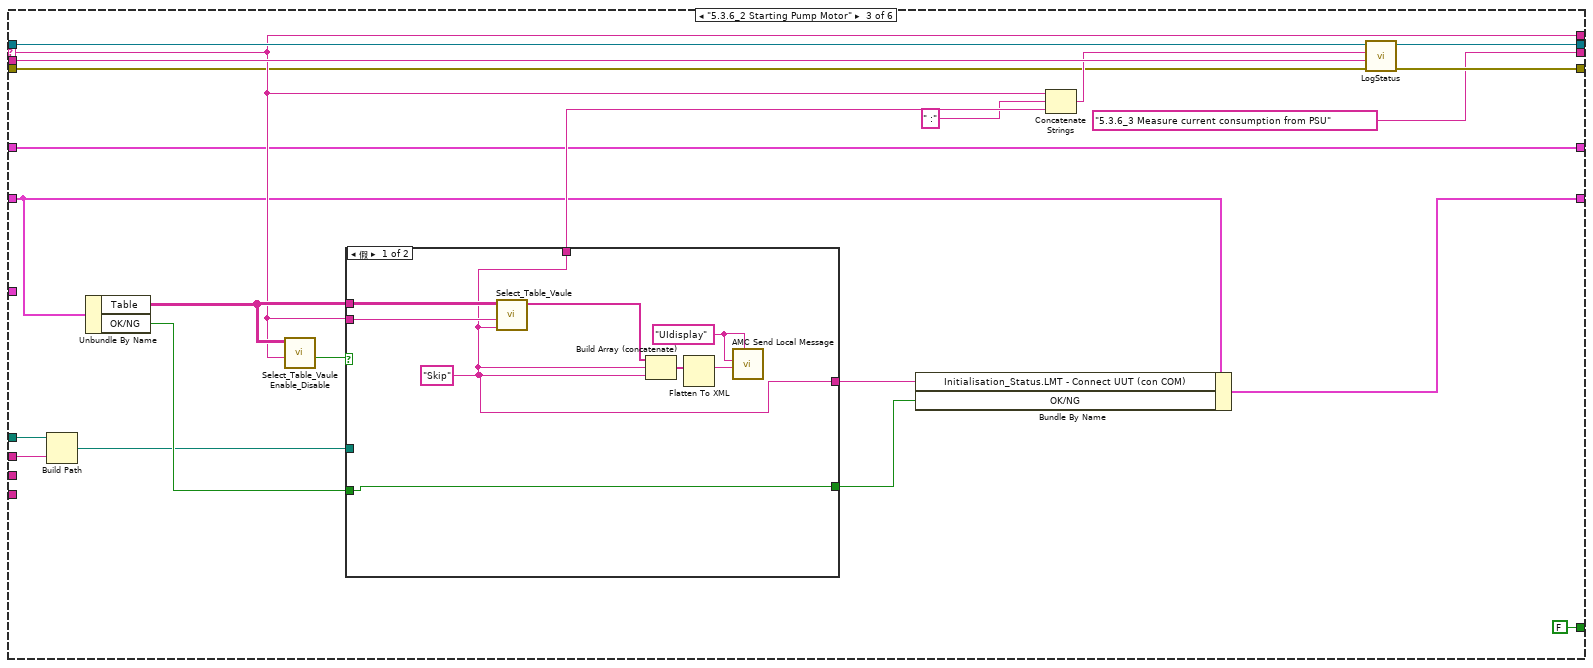
[diagram p6: hidden frame]
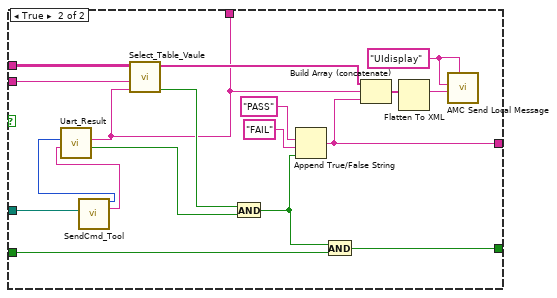
[diagram p7: hidden frame]
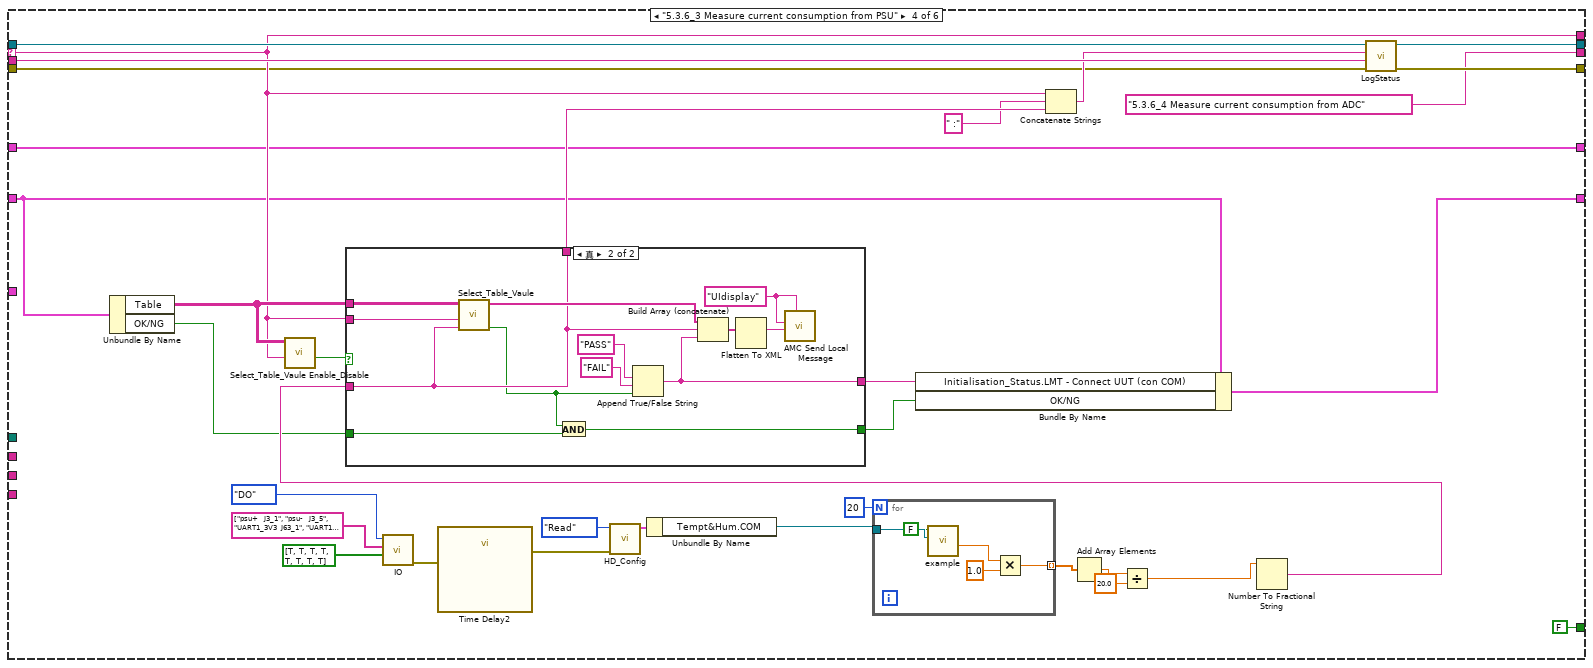
[diagram p8: hidden frame]
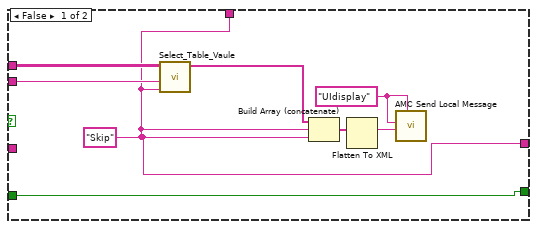
[diagram p9: hidden frame]
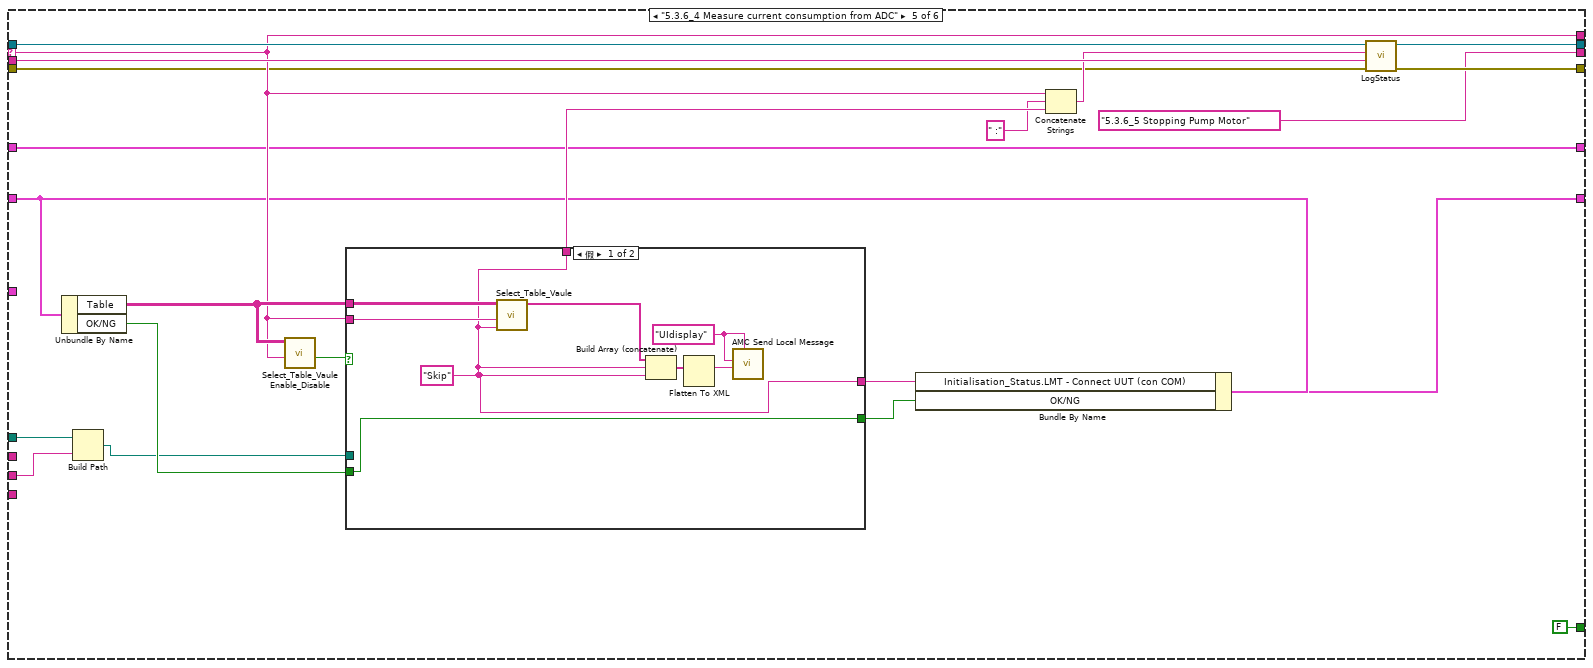
[diagram p10: hidden frame]
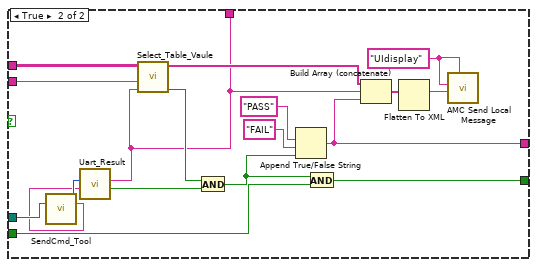
[diagram p11: hidden frame]
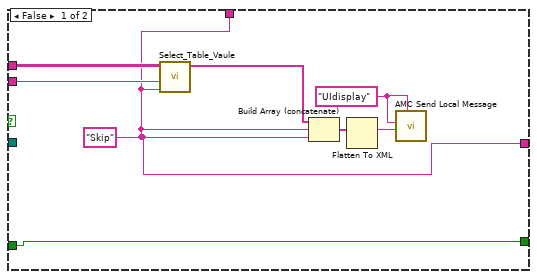
[diagram p12: hidden frame]
diagram:
  (unwired) "5.3.6_4 Stopping Pump Motor"
  (unwired) string[][] [["5.3.1_1 Set DC Power Supply", "", "NC", "Enable", "", "", ""], ["5.3.1_2 Measure current from DC Power Supply", "mA", "GELE", "Enable", "50", "", "550"], ["5.3.2_1 Send Get VP and SC Version", "", "NC", "Enable", "", "", ""], ["5.3.2_2 Stop Get VP and SC Version", "", "NC", "Enable", "", "", ""], ["5.3.3_1 Starting LED Test", "", "NC", "Enable", "", "Pass", ""], ["5.3.3_2 Operator to manually judge each LED", "", "NC", "Enable", "", "", ""], ["5.3.4_1 Self test", "", "NC", "Enable", "", "", ""], ["5.3.4_3 GetResponse", "", "NC", "Enable", "", "Pass", ""], ["5.3.5_1 Connect dummy brush motor to UUT", "", "NC", "Enable", "", "", ""], ["5.3.5_2 Starting Brush Motor in intensity 3", "", "Equal", "Enable", "", "3", ""], ["5.3.5_3 Measure current consumption from DMM; Intensity 3", "A", "GELE", "Enable", "0.209", "", "0.231"], ["5.3.5_4 Measure current consumption from ADC; Intensity 3", "", "NC", "Enable", "", "", ""], ["5.3.5_5 Starting Brush Motor in intensity 2", "", "Equal", "Enable", "", "2", ""], ["5.3.5_6 Measure current consumption from DMM; Intensity 2", "", "NC", "Enable", "TBC", "", "TBC"], ["5.3.5_7 Measure current consumption from ADC; Intensity 2", "", "NC", "Enable", "", "", ""], ["5.3.5_8 Starting Brush Motor in intensity 1", "", "Equal", "Enable", "", "1", ""], ["5.3.5_9 Measure current consumption from DMM; Intensity 1", "", "NC", "Enable", "TBC", "", "TBC"], ["5.3.5_10 Measure current consumption from ADC; Intensity 1", "", "NC", "Enable", "", "", ""], ["5.3.5_11 Stopping Brush Motor", "", "Equal", "Enable", "", "0", ""], ["5.3.6_1 Connect dummy pump motor to UUT", "", "NC", "Enable", "", "", ""], ["5.3.6_2 Starting Pump Motor", "", "Equal", "Enable", "", "1", ""], ["5.3.6_3 Measure current consumption from DMM", "A", "GELE", "Enable", "0.9025", "", "0.9975"], ["5.3.6_4 Measure current consumption from ADC", "", "NC", "Enable", "", "", ""], ["5.3.6_5 Stopping Pump Motor", "", "Equal", "Enable", "", "0", ""], ["5.3.7_1 MAC Address reading", "", "NC", "Enable", "", "", ""]] ("Table")
  (unwired) string[] ["5.3.1_1 Set DC Power Supply", "5.3.1_2 Measure current from DC Power Supply", "5.3.2_1 Send Get VP and SC Version", "5.3.2_2 Stop Get VP and SC Version", "5.3.3_1 Starting LED Test", "5.3.3_2 Operator to manually judge each LED", "5.3.4_1 Self test", "5.3.4_3 GetResponse", "5.3.5_1 Connect dummy brush motor to UUT", "5.3.5_2 Starting Brush Motor in intensity 3", "5.3.5_3 Measure current consumption from DMM; Intensity 3", "5.3.5_4 Starting Brush Motor in intensity 2", "5.3.5_5 Measure current consumption from DMM; Intensity 2", "5.3.5_6 Starting Brush Motor in intensity 1", "5.3.5_7 Measure current consumption from DMM; Intensity 1", "5.3.5_8 Stopping Brush Motor", "5.3.6_1 Connect dummy pump motor to UUT", "5.3.6_2 Starting Pump Motor", "5.3.6_3 Measure current consumption from DMM", "5.3.6_4 Stopping Pump Motor", "5.3.7_1 MAC Address reading"] ("subarray")
  n1 = Unbundle By Name(".batCMD") -> ("Starting  Pump Motor.bat"=w4:string, "Pump_ADC.bat"=w3:string, "Stopping  Pump Motor.bat"=w2:string)
  n2 = call "1-BasePath.vi"("Step"=enum16{"Initial", "Write", "Read"}."Read") -> ("Path Out"=w6:path)  [unwired: 9 in, 1 out]
  n3 = Flush Queue(queue="Message Queue out") -> (queue out=w14:T5)  [unwired: 1 in, 2 out]
  n4 = Build Path(base path=w6, name or relative path="Tool") -> (appended path=w5:path)
  n5 = call "AMC Send Local Message.vi"("error in (no error)"="error in (no error)", "Message Name"="5.3.6_1 Connect dummy pump motor to UUT", "Message Queue in"=w14) -> ("error out"=w18:errorcluster, "Message Queue out"=w19:T5)  [unwired: 7 in]
  n6 = while {
    tunnel: w19 -> [w54]
    tunnel: [w50] -> w13
    tunnel: w18 -> [w48]
    tunnel: [w45] -> w12
    shift-right: [w41] -> w15
    shift-left: "?" -> [w42]
    tunnel: "AllControls In" -> [w31]
    shift-right: [w29] -> w9
    shift-left: "Data in" -> [w30]
    tunnel: w5 -> [w25]
    tunnel: w4 -> [w24]
    tunnel: w3 -> [w23]
    tunnel: w2 -> [w22]
    stop <- w34 stop-if-true
    n7 = Wait (ms)(milliseconds to wait=u32 1 ("等待时间（毫秒）")) -> ()  [unwired: 1 out]
    n8 = call "AMC Read Next Message.vi"("error in (no error)"=w48, "timeout (1ms)"=100, "Message Queue in"=w54) -> ("error out"=w47:errorcluster, "Message Value"=w39:string, "Message Name"=w52:string, "Message Queue out"=w53:T5)  [unwired: 1 in, 4 out]
    n9 = case shown="\"5.3.6_5 Stopping Pump Motor\"" w52 {
      selector: w52 -> [_ w74 w124 w182 w229 w276]
      tunnel: w53 -> [w58 w79 w129 w187 w234 w281]
      tunnel: [w58 w79 w129 w187 w234 w281] -> w51
      tunnel: w47 -> [w57 w73 w123 w181 w228 w275]
      tunnel: [w57 w78 w128 w186 w233 w280] -> w46
      tunnel: [_ FALSE ("GRR") FALSE ("GRR") FALSE ("GRR") FALSE ("GRR") TRUE ("GRR")] -> w35
      tunnel: w42 -> [w56 w69 w119 w177 w224 w272]
      tunnel: [w56 w69 w119 w177 w224 w272] -> w41
      tunnel: w39 -> [_ w77 w127 w185 w232 w279]
      tunnel: [_ w74 w124 w182 w229 w276] -> w38
      tunnel: [_ "5.3.6_2 Starting Pump Motor" "5.3.6_3 Measure current consumption from PSU" "5.3.6_4 Measure current consumption from ADC" "5.3.6_5 Stopping Pump Motor" "Disconnect_UUT"] -> w40
      tunnel: w31 -> [_ _ _ _ _ _]
      tunnel: w30 -> [w55 w68 w118 w176 w223 w271]
      tunnel: [w55 w67 w117 w175 w222 w270] -> w29
      tunnel: w25 -> [_ _ w114 _ w219 w266]
      tunnel: w24 -> [_ _ w113 _ _ _]
      tunnel: w23 -> [_ _ _ _ w218 _]
      tunnel: w22 -> [_ _ _ _ _ w267]
      frame "假", Default {
      }
      frame "5.3.6_1 Connect pump motor to UUT" {
        n10 = disable-structure shown="禁用" {
          disable-tunnel: [w82 _] -> w61
          disable-tunnel: [w81 _] -> w60
          disable-tunnel: [w80 _] -> w59
          frame Disabled {
            w80 = "Fail" ("F按钮名称（“取消”）")
            w81 = "Pass" ("T按钮名称（“确定”）")
            n11 = Two Button Dialog(message="Connect pump motor?" ("消息"), 1:w80, 2:w81) -> (T button?=w82:bool)
          }
          frame Enabled {
          }
        }
        n12 = Unbundle By Name(w68) -> ("Table"=w75:string[][], "OK/NG"=w64:bool)
        n13 = call "Select_Table_Vaule Enable_Disable.vi"("Action"=w74, "Table"=w75) -> ("Enable"=w71:bool)  [unwired: 8 in, 1 out]
        n14 = case shown="假" w71 {
          tunnel: [w85 w95] -> w72
          tunnel: w75 -> [w87 w102]
          tunnel: w74 -> [w86 w101]
          tunnel: [w85 w100] -> w66
          tunnel: w64 -> [w84 w99]
          tunnel: [w84 w98] -> w63
          tunnel: w61 -> [_ w93]
          tunnel: w60 -> [_ w97]
          tunnel: w59 -> [_ w96]
          frame False {
            w91 = "UIdisplay" ("Process (\"\" - local)")
            w85 = "Skip" ("Action")
            n15 = call "Select_Table_Vaule.vi"("Vaule"=w85, "Action"=w86, "Table"=w87) -> ("vaule"=w88:string[])  [unwired: 7 in, 1 out]
            n16 = Build Array (concatenate)(w88, w85, w85) -> (w90:string[])
            n17 = Flatten To XML(anything=w90) -> (xml string=w89:string)
            n18 = call "AMC Send Local Message.vi"("Process (\"\" - local)"=w91, "Message Value"=w89, "Message Name"=w91) -> ()  [unwired: 7 in, 2 out]
          }
          frame True {
            w107 = "UIdisplay" ("Process (\"\" - local)")
            n19 = Select(t=w97, s=w93, f=w96) -> (s? t:f=w95:string)
            n20 = call "Select_Table_Vaule.vi"("Vaule"=w95, "Action"=w101, "Table"=w102) -> ("Result"=w94:bool, "vaule"=w108:string[])  [unwired: 7 in]
            n21 = And(x=w94, y=w93) -> (x .and. y?=w92:bool)
            n22 = And(x=w92, y=w99) -> (x .and. y?=w98:bool)
            n23 = Append True/False String(1:w92, 2:"FAIL" ("真字符串"), 3:"PASS" ("真字符串")) -> (0:w100:string)  [unwired: 1 in]
            n24 = Build Array (concatenate)(w108, w95, w100) -> (w106:string[])
            n25 = Flatten To XML(anything=w106) -> (xml string=w105:string)
            n26 = call "AMC Send Local Message.vi"("Process (\"\" - local)"=w107, "Message Value"=w105, "Message Name"=w107) -> ()  [unwired: 7 in, 2 out]
          }
        }
        n27 = Bundle By Name(cluster=w68, "Initialisation_Status.LMT - Connect UUT (con COM)"=w66, "OK/NG"=w63) -> (w67:T2)
        n28 = Concatenate Strings(w74, " :", w72) -> (w76:string)
        n29 = call "LogStatus.vi"("error in (no error)"=w73, "last message"=w77, "message"=w76) -> ("error  out"=w78:errorcluster)  [unwired: 8 in]
      }
      frame "5.3.6_2 Starting Pump Motor" {
        n30 = Build Path(base path=w114, name or relative path=w113) -> (appended path=w109:path)
        n31 = Unbundle By Name(w118) -> ("Table"=w125:string[][], "OK/NG"=w112:bool)
        n32 = call "Select_Table_Vaule Enable_Disable.vi"("Action"=w124, "Table"=w125) -> ("Enable"=w121:bool)  [unwired: 8 in, 1 out]
        n33 = case shown="假" w121 {
          tunnel: [w131 w143] -> w122
          tunnel: w125 -> [w133 w149]
          tunnel: w124 -> [w132 w148]
          tunnel: [w131 w147] -> w116
          tunnel: w112 -> [w130 w141]
          tunnel: [w130 w144] -> w111
          tunnel: w109 -> [_ w140]
          frame False {
            w137 = "UIdisplay" ("Process (\"\" - local)")
            w131 = "Skip" ("Action")
            n34 = call "Select_Table_Vaule.vi"("Vaule"=w131, "Action"=w132, "Table"=w133) -> ("vaule"=w134:string[])  [unwired: 7 in, 1 out]
            n35 = Build Array (concatenate)(w134, w131, w131) -> (w136:string[])
            n36 = Flatten To XML(anything=w136) -> (xml string=w135:string)
            n37 = call "AMC Send Local Message.vi"("Process (\"\" - local)"=w137, "Message Value"=w135, "Message Name"=w137) -> ()  [unwired: 7 in, 2 out]
          }
          frame True {
            w154 = "UIdisplay" ("Process (\"\" - local)")
            n38 = call "SendCmd_Tool.vi"("path_bat"=w140) -> ("return code"=w139:i32, "Other"=w138:string)  [unwired: 6 in, 7 out]
            n39 = call "Uart_Result.vi"("input"=w138, "return code"=w139) -> ("Command Sucess"=w142:bool, "return_result"=w143:string)  [unwired: 8 in]
            n40 = call "Select_Table_Vaule.vi"("Vaule"=w143, "Action"=w148, "Table"=w149) -> ("Result"=w146:bool, "vaule"=w155:string[])  [unwired: 7 in]
            n41 = And(x=w146, y=w142) -> (x .and. y?=w145:bool)
            n42 = Append True/False String(1:w145, 2:"FAIL" ("真字符串"), 3:"PASS" ("真字符串")) -> (0:w147:string)  [unwired: 1 in]
            n43 = And(x=w145, y=w141) -> (x .and. y?=w144:bool)
            n44 = Build Array (concatenate)(w155, w143, w147) -> (w153:string[])
            n45 = Flatten To XML(anything=w153) -> (xml string=w152:string)
            n46 = call "AMC Send Local Message.vi"("Process (\"\" - local)"=w154, "Message Value"=w152, "Message Name"=w154) -> ()  [unwired: 7 in, 2 out]
          }
        }
        n47 = Bundle By Name(cluster=w118, "Initialisation_Status.LMT - Connect UUT (con COM)"=w116, "OK/NG"=w111) -> (w117:T2)
        n48 = Concatenate Strings(w124, " :", w122) -> (w126:string)
        n49 = call "LogStatus.vi"("error in (no error)"=w123, "last message"=w127, "message"=w126) -> ("error  out"=w128:errorcluster)  [unwired: 8 in]
      }
      frame "5.3.6_3 Measure current consumption from PSU" {
        n50 = Unbundle By Name(w176) -> ("Table"=w183:string[][], "OK/NG"=w158:bool)
        n51 = call "Select_Table_Vaule Enable_Disable.vi"("Action"=w182, "Table"=w183) -> ("Enable"=w179:bool)  [unwired: 8 in, 1 out]
        n52 = call "IO.vi"("DO DATA"=bool[] [TRUE, TRUE, TRUE, TRUE, TRUE, TRUE, TRUE, TRUE], "IO Name"=string[] ["psu+   J3_1", "psu-   J3_5", "UART1_3V3  J63_1", "UART1_TX   J63_5", "UART1_RX   J63_6", "UART1_GND  J63_10", "PSU S+ J3_1", "PSU S- J3_5"], "IO?"=enum16{"DI", "DO"}."DO") -> ("error out"=w169:errorcluster)  [unwired: 7 in, 1 out]
        n53 = call "Time Delay2"("error in (no error)"=w169) -> ("error out"=w166:errorcluster)  [unwired: 10 in]
        n54 = call "HD_Config.vi"("error in (no error)"=w166, "Step"=enum16{"Initial", "Write", "Read"}."Read") -> ("HD Config out"=w168:T6)  [unwired: 8 in, 1 out]
        n55 = Unbundle By Name(w168) -> ("Tempt&Hum.COM"=w160:refnum<visa-resource-name>)
        n56 = for {
          N: 20 -> [_]
          tunnel: w160 -> [w192]
          tunnel: [w188] -> w163 mode=indexing
          n57 = call <instrlib>:"example.vi"("VISA resource name"=w192, "FLAG"=FALSE) -> ("Actual Current Level (A)"=w189:dbl)  [unwired: 6 in, 3 out]
          n58 = Multiply(x=w189, y=1.0) -> (x*y=w188:dbl)
        }
        n59 = Add Array Elements(numeric array=w163) -> (sum=w162:dbl)
        n60 = Divide(x=w162, y=20.0) -> (x/y=w159:dbl)
        n61 = Number To Fractional String(number=w159) -> (F-format string=w165:string)  [unwired: 3 in]
        n62 = case shown="真" w179 {
          tunnel: [w194 w205] -> w180
          tunnel: w183 -> [w196 w207]
          tunnel: w182 -> [w195 w206]
          tunnel: w165 -> [_ w205]
          tunnel: [w194 w204] -> w174
          tunnel: w158 -> [w193 w202]
          tunnel: [w193 w201] -> w157
          frame False {
            w200 = "UIdisplay" ("Process (\"\" - local)")
            w194 = "Skip" ("Action")
            n63 = call "Select_Table_Vaule.vi"("Vaule"=w194, "Action"=w195, "Table"=w196) -> ("vaule"=w197:string[])  [unwired: 7 in, 1 out]
            n64 = Build Array (concatenate)(w197, w194, w194) -> (w199:string[])
            n65 = Flatten To XML(anything=w199) -> (xml string=w198:string)
            n66 = call "AMC Send Local Message.vi"("Process (\"\" - local)"=w200, "Message Value"=w198, "Message Name"=w200) -> ()  [unwired: 7 in, 2 out]
          }
          frame True {
            w212 = "UIdisplay" ("Process (\"\" - local)")
            n67 = call "Select_Table_Vaule.vi"("Vaule"=w205, "Action"=w206, "Table"=w207) -> ("Result"=w203:bool, "vaule"=w213:string[])  [unwired: 7 in]
            n68 = And(x=w203, y=w202) -> (x .and. y?=w201:bool)
            n69 = Append True/False String(1:w203, 2:"FAIL" ("真字符串"), 3:"PASS" ("真字符串")) -> (0:w204:string)  [unwired: 1 in]
            n70 = Build Array (concatenate)(w213, w205, w204) -> (w211:string[])
            n71 = Flatten To XML(anything=w211) -> (xml string=w210:string)
            n72 = call "AMC Send Local Message.vi"("Process (\"\" - local)"=w212, "Message Value"=w210, "Message Name"=w212) -> ()  [unwired: 7 in, 2 out]
          }
        }
        n73 = Bundle By Name(cluster=w176, "Initialisation_Status.LMT - Connect UUT (con COM)"=w174, "OK/NG"=w157) -> (w175:T2)
        n74 = Concatenate Strings(w182, " :", w180) -> (w184:string)
        n75 = call "LogStatus.vi"("error in (no error)"=w181, "last message"=w185, "message"=w184) -> ("error  out"=w186:errorcluster)  [unwired: 8 in]
      }
      frame "5.3.6_4 Measure current consumption from ADC" {
        n76 = Unbundle By Name(w223) -> ("Table"=w230:string[][], "OK/NG"=w217:bool)
        n77 = Build Path(base path=w219, name or relative path=w218) -> (appended path=w214:path)
        n78 = call "Select_Table_Vaule Enable_Disable.vi"("Action"=w229, "Table"=w230) -> ("Enable"=w226:bool)  [unwired: 8 in, 1 out]
        n79 = case shown="假" w226 {
          tunnel: [w236 w247] -> w227
          tunnel: w230 -> [w238 w254]
          tunnel: w229 -> [w237 w253]
          tunnel: [w236 w252] -> w221
          tunnel: w217 -> [w235 w249]
          tunnel: [w235 w248] -> w216
          tunnel: w214 -> [_ w245]
          frame False {
            w242 = "UIdisplay" ("Process (\"\" - local)")
            w236 = "Skip" ("Action")
            n80 = call "Select_Table_Vaule.vi"("Vaule"=w236, "Action"=w237, "Table"=w238) -> ("vaule"=w239:string[])  [unwired: 7 in, 1 out]
            n81 = Build Array (concatenate)(w239, w236, w236) -> (w241:string[])
            n82 = Flatten To XML(anything=w241) -> (xml string=w240:string)
            n83 = call "AMC Send Local Message.vi"("Process (\"\" - local)"=w242, "Message Value"=w240, "Message Name"=w242) -> ()  [unwired: 7 in, 2 out]
          }
          frame True {
            w259 = "UIdisplay" ("Process (\"\" - local)")
            n84 = call "SendCmd_Tool.vi"("path_bat"=w245) -> ("return code"=w244:i32, "Other"=w243:string)  [unwired: 6 in, 7 out]
            n85 = call "Uart_Result.vi"("input"=w243, "return code"=w244) -> ("Command Sucess"=w246:bool, "return_result"=w247:string)  [unwired: 8 in]
            n86 = call "Select_Table_Vaule.vi"("Vaule"=w247, "Action"=w253, "Table"=w254) -> ("Result"=w251:bool, "vaule"=w260:string[])  [unwired: 7 in]
            n87 = And(x=w251, y=w246) -> (x .and. y?=w250:bool)
            n88 = Append True/False String(1:w250, 2:"FAIL" ("真字符串"), 3:"PASS" ("真字符串")) -> (0:w252:string)  [unwired: 1 in]
            n89 = And(x=w250, y=w249) -> (x .and. y?=w248:bool)
            n90 = Build Array (concatenate)(w260, w247, w252) -> (w258:string[])
            n91 = Flatten To XML(anything=w258) -> (xml string=w257:string)
            n92 = call "AMC Send Local Message.vi"("Process (\"\" - local)"=w259, "Message Value"=w257, "Message Name"=w259) -> ()  [unwired: 7 in, 2 out]
          }
        }
        n93 = Bundle By Name(cluster=w223, "Initialisation_Status.LMT - Connect UUT (con COM)"=w221, "OK/NG"=w216) -> (w222:T2)
        n94 = Concatenate Strings(w229, " :", w227) -> (w231:string)
        n95 = call "LogStatus.vi"("error in (no error)"=w228, "last message"=w232, "message"=w231) -> ("error  out"=w233:errorcluster)  [unwired: 8 in]
      }
      frame "5.3.6_5 Stopping Pump Motor" {
        (unwired) "5.3.7 MAC Address reading"
        n96 = Unbundle By Name(w271) -> ("Table"=w277:string[][], "OK/NG"=w265:bool)
        n97 = Build Path(base path=w266, name or relative path=w267) -> (appended path=w261:path)
        n98 = call "Select_Table_Vaule Enable_Disable.vi"("Action"=w276, "Table"=w277) -> ("Enable"=w273:bool)  [unwired: 8 in, 1 out]
        n99 = case shown="真" w273 {
          tunnel: [w283 w293] -> w274
          tunnel: w277 -> [w285 w301]
          tunnel: w276 -> [w284 w300]
          tunnel: [w283 w299] -> w269
          tunnel: w265 -> [w282 w296]
          tunnel: [w282 w295] -> w264
          tunnel: w261 -> [_ w292]
          frame False {
            w289 = "UIdisplay" ("Process (\"\" - local)")
            w283 = "Skip" ("Action")
            n100 = call "Select_Table_Vaule.vi"("Vaule"=w283, "Action"=w284, "Table"=w285) -> ("vaule"=w286:string[])  [unwired: 7 in, 1 out]
            n101 = Build Array (concatenate)(w286, w283, w283) -> (w288:string[])
            n102 = Flatten To XML(anything=w288) -> (xml string=w287:string)
            n103 = call "AMC Send Local Message.vi"("Process (\"\" - local)"=w289, "Message Value"=w287, "Message Name"=w289) -> ()  [unwired: 7 in, 2 out]
          }
          frame True {
            w306 = "UIdisplay" ("Process (\"\" - local)")
            n104 = call "SendCmd_Tool.vi"("path_bat"=w292) -> ("return code"=w291:i32, "Other"=w290:string)  [unwired: 6 in, 7 out]
            n105 = call "Uart_Result.vi"("input"=w290, "return code"=w291) -> ("Command Sucess"=w294:bool, "return_result"=w293:string)  [unwired: 8 in]
            n106 = call "Select_Table_Vaule.vi"("Vaule"=w293, "Action"=w300, "Table"=w301) -> ("Result"=w298:bool, "vaule"=w307:string[])  [unwired: 7 in]
            n107 = And(x=w298, y=w294) -> (x .and. y?=w297:bool)
            n108 = Append True/False String(1:w297, 2:"FAIL" ("真字符串"), 3:"PASS" ("真字符串")) -> (0:w299:string)  [unwired: 1 in]
            n109 = And(x=w297, y=w296) -> (x .and. y?=w295:bool)
            n110 = Build Array (concatenate)(w307, w293, w299) -> (w305:string[])
            n111 = Flatten To XML(anything=w305) -> (xml string=w304:string)
            n112 = call "AMC Send Local Message.vi"("Process (\"\" - local)"=w306, "Message Value"=w304, "Message Name"=w306) -> ()  [unwired: 7 in, 2 out]
          }
        }
        n113 = Bundle By Name(cluster=w271, "Initialisation_Status.LMT - Connect UUT (con COM)"=w269, "OK/NG"=w264) -> (w270:T2)
        n114 = Concatenate Strings(w276, " :", w274) -> (w278:string)
        n115 = call "LogStatus.vi"("error in (no error)"=w275, "last message"=w279, "message"=w278) -> ("error  out"=w280:errorcluster)  [unwired: 8 in]
      }
    }
    n116 = call "Stop.vi"("Step"=enum16{"Initial", "Write", "Read"}."Read") -> ("Stop Out"=w33:bool)  [unwired: 9 in, 1 out]
    n117 = call "Exit.vi"("Step"=enum16{"Initial", "Write", "Read"}."Read" ("step")) -> ("Exit Out"=w32:bool)  [unwired: 9 in, 1 out]
    n118 = call "6-AlarmStatus.vi"("Step"=enum16{"Initial", "Write", "Read"}."Read") -> ("AlarmValue Out"=w27:bool[])  [unwired: 9 in, 1 out]
    n119 = Or Array Elements(Boolean array=w27) -> (logical OR=w26:bool)
    n120 = call "AMC Run Step.vi"("Message Queue In"=w51, "Message Name"=w40, "Message Value"=w38, "error in (no error)"=w46, "Mli/Sig"=FALSE) -> ("Message Queue Out"=w50:T5, "error out"=w45:errorcluster)  [unwired: 13 in]
    n121 = Compound Arithmetic op=OR(w35, w33, w32, w26) -> (w34:bool)
  }
  "Message Queue Out" <- w13
  "error out" <- w12
  "Data" <- w15
  "Data out" <- w9
